vi "poly_control_value_from_name_caller_multi.vi"(8 "error in (no error)":errorcluster, 9 "control names":string[](array[string]), 10 "name of caller in (your caller)":string) -> (0 "error out":errorcluster, 1 "Values":variant[](array[variant]), 4 "found?":bool[](array[boolean]), 5 "ctrl refs":refnum<vi>[](array[refnum]))   [LabVIEW 2015]
uses:
  poly_ref_tools_eco_plus.vi
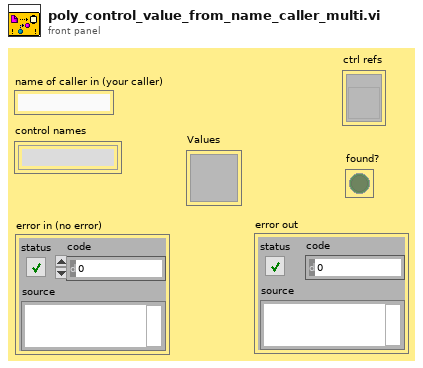
[diagram p1: front panel]
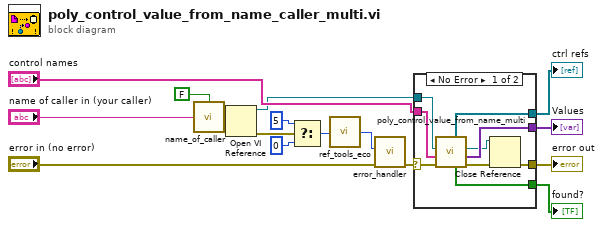
[diagram p0: block diagram]
diagram:
  n1 = call "name_of_caller.vi"("is in inlined vi? (F)"=FALSE, "name of caller in"="name of caller in (your caller)") -> ("name of caller out"=w10:string)  [unwired: 2 in]
  n2 = Open VI Reference(vi path=w10) -> (vi reference=w12:refnum<vi>, error out=w3:errorcluster)  [unwired: 5 in]
  n3 = Select(t=5, s=w3, f=0) -> (s? t:f=w5:i32)
  n4 = call-poly "ref_tools_eco.vi"("code (w/out eco)"=w5) -> ("code (+ eco)"=w4:i32)  [unwired: 4 in]
  n5 = call "error_handler.vi"("error in (no error)"="error in (no error)", "code (0 = no error)"=w4) -> ("error out"=w1:errorcluster)  [unwired: 8 in, 1 out]
  n6 = case shown="No Error" w1 {
    selector: w1 -> [w17 w26]
    tunnel: "control names" -> [w25 _]
    tunnel: [w24 _] -> w15
    tunnel: [w23 _] -> w14
    tunnel: [w22 _] -> w13
    tunnel: w12 -> [w19 _]
    tunnel: [w18 w26] -> w11
    frame No Error {
      n7 = call "poly_control_value_from_name_multi.vi"("error in (no error)"=w17, "control names"=w25, "vi ref"=w19) -> ("error out"=w21:errorcluster, "Values"=w24:variant[], "vi ref dup"=w20:refnum<vi>, "found?"=w22:bool[], "ctrl refs"=w23:refnum<vi>[])  [unwired: 4 in]
      n8 = Close Reference(reference=w20, error in (no error)=w21) -> (error out=w18:errorcluster)
    }
    frame Error {
    }
  }
  "error out" <- w11
  "Values" <- w15
  "ctrl refs" <- w14
  "found?" <- w13
